vi "Aim Turret.vi"(0 "Setpoint (testing purposes only)":dbl, 1 "Goal Detected":bool=TRUE, 2 "Override?":bool, 3 "Override Setpoint":dbl, 4 "MotorControlDevRef":T2={"DeviceStatus"={"status"=FALSE, "code"=0, "source"=""}, "Type"=enum."CANTalonSRX", "PWM"={"PWM Channel"=enum."PWM 1", "DeadBand"={"Name"="", "maxPositivePwm"=0, "minPositivePwm"=0, "centerPwm"=0, "maxNegativePwm"=0, "minNegativePwm"=0, "angularRange"=0}}, "CAN"={"Device Number"=11, "Control Mode"=enum."Percent VBus", "Semaphore"=refnum, "Max Vout"=12.0, "TalonSRX Control Mode"=enum."Position"}, "Invert"=TRUE}, 5 "Goal Angle Degrees 0=straight ahead":dbl=0.37665367540620964, 6 "Yaw (degrees 0 = straight ahead gets larger clockwise)":dbl=-20.33, 7 "Sensor Position (degrees)":dbl=20.326171875, 9 "Softlimit":dbl=145.0 format="%#_13g") -> (14 "Output":dbl=20.702825550406203, 15 "Finished?":bool=TRUE, 18 "Override Still Enabled":bool)   [LabVIEW 2015]
uses:
  <vilib>/Rock Robotics/WPI/MotorControl/WPI_MotorControlDeviceRef.ctl
  <vilib>/Rock Robotics/WPI/MotorControl/WPI_MotorControlType.ctl
  <vilib>/Rock Robotics/SystemInterfaces/DIO/FPGA_DIOPWMChannel.ctl
  <vilib>/Rock Robotics/WPI/PWM/WPI_PWMDeadband.ctl
  <vilib>/Rock Robotics/WPI/CAN/Jaguar/SubVIs/WPI_CANJaguar_ControlMode.ctl
  <vilib>/Rock Robotics/WPI/CAN/TalonSRX/WPI_CANTalonSRX_APIControlMode.ctl
  Robot Global Data.vi
panel:
  in  "Turret PID (position) Long Distance Seek":T1={"P"=0.21, "I"=0.0021, "D"=3.0, "F"=0.0, "I Zone"=1200.0}
  in  "Turret PID (position) Short distance seek":T1={"P"=0.0015, "I"=0.0035, "D"=0.0, "F"=0.0, "I Zone"=1400.0}
  in  "Delay (ms)":i32=750
  in  "Turret revolutions per shooter revolution":dbl=15.0
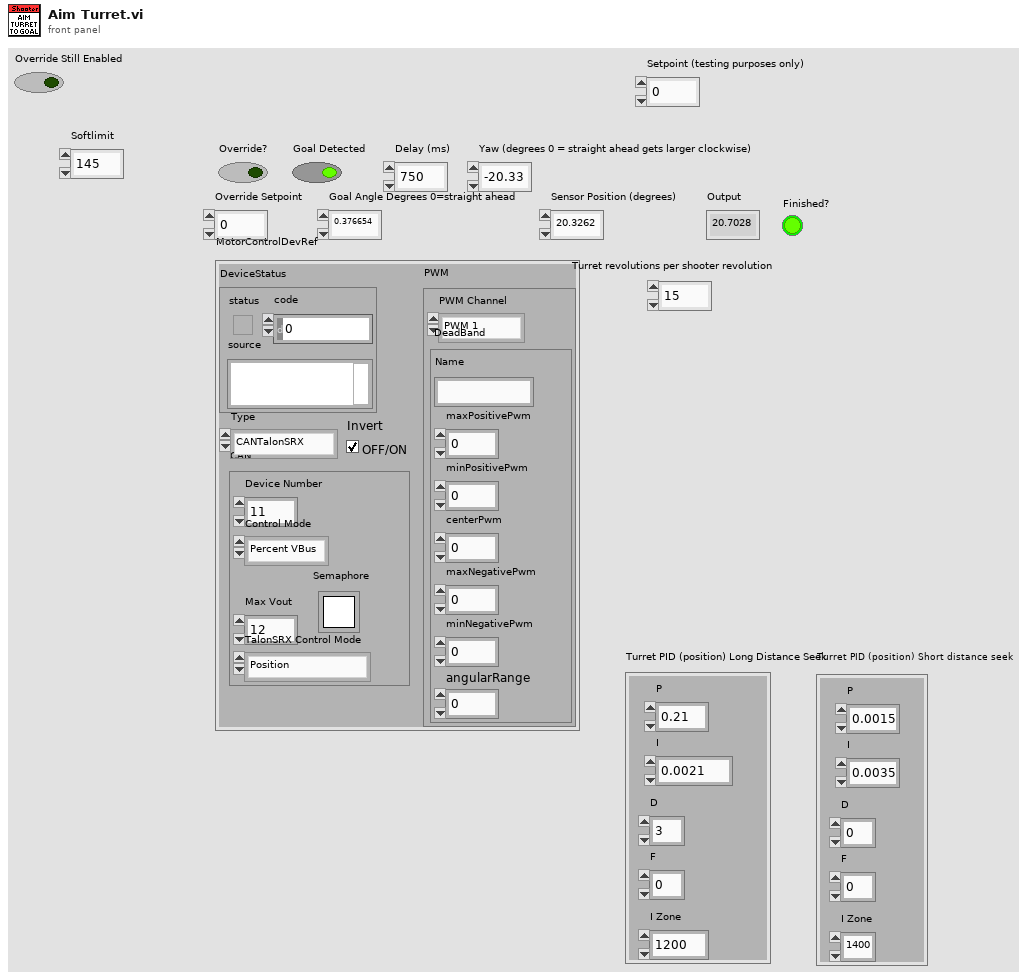
[diagram p1: front panel]
types:
  T1 = cluster{"P":dbl, "I":dbl, "D":dbl, "F":dbl, "I Zone":dbl}
  T2 = typedef "WPI_MotorControlDeviceRef.ctl" = cluster{"DeviceStatus":errorcluster, "Type":T3, "PWM":cluster{"PWM Channel":T4, "DeadBand":T5}, "CAN":cluster{"Device Number":u8, "Control Mode":T6, "Semaphore":T7, "Max Vout":dbl, "TalonSRX Control Mode":T8}, "Invert":bool}
  T3 = typedef "WPI_MotorControlType.ctl" = enum16{"PWM", "CAN", "CANTalonSRX"}
  T4 = typedef "FPGA_DIOPWMChannel.ctl" = enum8{"PWM 0", "PWM 1", "PWM 2", "PWM 3", "PWM 4", "PWM 5", "PWM 6", "PWM 7", "PWM 8", "PWM 9", "PWM MXP 0", "PWM MXP 1", "PWM MXP 2", "PWM MXP 3", "PWM MXP 4", "PWM MXP 5", "PWM MXP 6", "PWM MXP 7", "PWM MXP 8", "PWM MXP 9", "Invalid"}
  T5 = typedef "WPI_PWMDeadband.ctl" = cluster{"Name":string, "maxPositivePwm":i32, "minPositivePwm":i32, "centerPwm":i32, "maxNegativePwm":i32, "minNegativePwm":i32, "angularRange":u16}
  T6 = typedef "WPI_CANJaguar_ControlMode.ctl" = enum8{"Percent VBus", "Current", "Speed", "Position", "Voltage"}
  T7 = typedef "Semaphore RefNum" = refnum<k1>
  T8 = typedef "WPI_CANTalonSRX_APIControlMode.ctl" = enum8{"Percent VBus", "Speed", "Position", "Slave", "Unchanged / Invalid", "Voltage Compensation", "Current", "Motion Profile"}
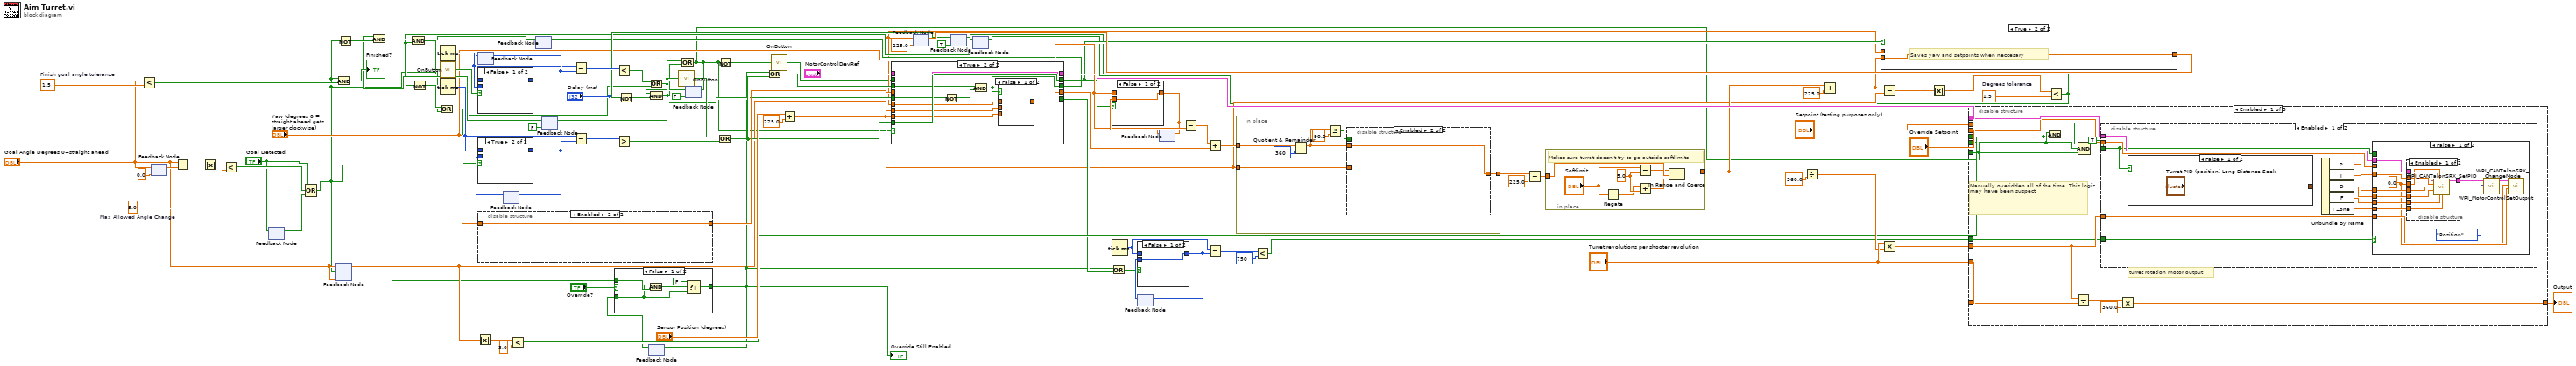
[diagram p0: block diagram]
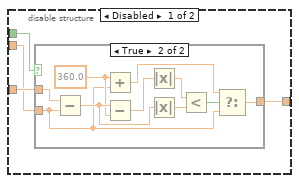
[diagram p4: hidden frame]
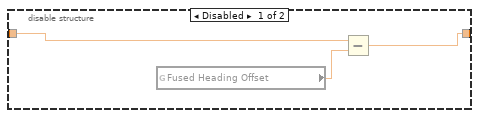
[diagram p6: hidden frame]
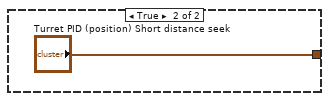
[diagram p10: hidden frame]
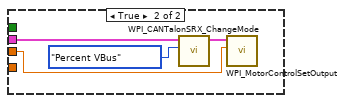
[diagram p12: hidden frame]
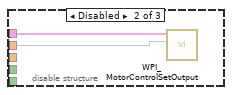
[diagram p14: hidden frame]
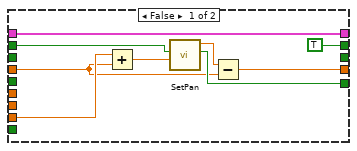
[diagram p17: hidden frame]
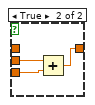
[diagram p18: hidden frame]
diagram:
  w11 = 5.0  # Max Allowed Angle Change
  w44 = 1.5  # Degrees tolerance
  w86 = 1.5  # Finish goal angle tolerance
  n1 = Less?(x="Goal Angle Degrees 0=straight ahead", y=w86) -> (x < y?=w85:bool)
  n2 = feedback-in #1("Goal Angle Degrees 0=straight ahead") -> ()
  n3 = feedback #1(0.0 ("Goal Angle Degrees 0=straight ahead")) -> (w15:dbl)
  n4 = Subtract(x="Goal Angle Degrees 0=straight ahead", y=w15) -> (x-y=w13:dbl)
  n5 = Absolute Value(x=w13) -> (abs(x)=w12:dbl)
  n6 = Less?(x=w12, y=w11) -> (x < y?=w4:bool)
  n7 = feedback-in #2("Goal Detected") -> ()
  n8 = feedback #2() -> (w5:bool)  [unwired: 1 in]
  n9 = Compound Arithmetic op=OR("Goal Detected", w4, w5) -> (w2:bool)
  n10 = feedback-in #3("Goal Angle Degrees 0=straight ahead", w2) -> ()
  n11 = feedback #3("Goal Angle Degrees 0=straight ahead") -> (w9:dbl)
  n12 = Not(x=w2) -> (.not. x?=w70:bool)
  n13 = Compound Arithmetic op=AND(w2, w85) -> (→"Finished?":bool)
  n14 = Tick Count (ms)() -> (millisecond timer value=w73:u32)
  n15 = Tick Count (ms)() -> (millisecond timer value=w79:u32)
  n16 = Absolute Value(x=w9) -> (abs(x)=w16:dbl)
  n17 = feedback #4() -> (w75:u32)  [unwired: 1 in]
  n18 = disable-structure shown="Enabled" {
    disable-tunnel: [w99 w100] -> w89
    disable-tunnel: "Yaw (degrees 0 = straight ahead gets larger clockwise)" -> [w97 w100]
    frame Disabled {
      n19 = global read "Robot Global Data.vi" "Fused Heading Offset"() -> (w98:dbl)
      n20 = Subtract(x=w97, y=w98) -> (x-y=w99:dbl)
    }
    frame Enabled {
    }
  }
  n21 = feedback #5() -> (w82:u32)  [unwired: 1 in]
  n22 = Less?(x=w16, y=3.0 ("x")) -> (x < y?=w31:bool)
  n23 = feedback #6() -> (w37:bool)  [unwired: 1 in]
  n24 = feedback #7(FALSE) -> (w69:bool)
  n25 = And(x=w69, y=w70) -> (x .and. y?=w68:bool)
  n26 = feedback #8() -> (w8:bool)  [unwired: 1 in]
  n27 = case shown="False" "Override?" {
    selector: "Override?" -> [_ w106]
    tunnel: [w101 w106] -> w6
    tunnel: w8 -> [w102 _]
    tunnel: w2 -> [w105 _]
    frame False {
      n28 = And(x=w102, y=w105) -> (x .and. y?=w104:bool)
      n29 = Select(t=FALSE, s=w104, f=w102) -> (s? t:f=w101:bool)
    }
    frame True {
    }
  }
  "Override Still Enabled" <- w6
  n30 = feedback-in #8(w6) -> ()
  n31 = feedback #9(FALSE) -> (w63:bool)
  n32 = Add(x="Sensor Position (degrees)", y=225.0) -> (x+y=w18:dbl)
  n33 = feedback #10(225.0) -> (w32:dbl)
  n34 = feedback #11(TRUE) -> (w64:bool)
  n35 = Not(x=w64) -> (.not. x?=w78:bool)
  n36 = And(x=w63, y=w78) -> (x .and. y?=w42:bool)
  n37 = feedback #12() -> (w40:bool)  [unwired: 1 in]
  n38 = And(x=w68, y=w40) -> (x .and. y?=w66:bool)
  n39 = Not(x=w40) -> (.not. x?=w39:bool)
  n40 = Or(x=w39, y=w37) -> (x .or. y?=w38:bool)
  n41 = call "OnButton.vi"("Button"=w66) -> ("Value"=w65:bool)  [unwired: 1 in]
  n42 = case shown="False" w65 {
    tunnel: [w107 w108] -> w74
    tunnel: w73 -> [_ w108]
    tunnel: w75 -> [w107 _]
    frame False {
    }
    frame True {
    }
  }
  n43 = feedback-in #4(w74) -> ()
  n44 = case shown="True" w38 {
    tunnel: [w109 w110] -> w81
    tunnel: w79 -> [_ w110]
    tunnel: w82 -> [w109 _]
    frame False {
    }
    frame True {
    }
  }
  n45 = feedback-in #5(w81) -> ()
  n46 = Subtract(x=w73, y=w74) -> (x-y=w76:u32)
  n47 = Subtract(x=w79, y=w81) -> (x-y=w83:u32)
  n48 = Less?(x=w76, y="Delay (ms)") -> (x < y?=w72:bool)
  n49 = Greater?(x=w83, y="Delay (ms)") -> (0:w80:bool)
  n50 = Or(x=w72, y=w2) -> (x .or. y?=w71:bool)
  n51 = feedback-in #7(w71) -> ()
  n52 = call "OnButton.vi"("Button"=w71) -> ("Value"=w77:bool)  [unwired: 1 in]
  n53 = Or(x=w71, y=w42) -> (x .or. y?=w1:bool)
  n54 = feedback-in #9(w1) -> ()
  n55 = Or(x=w77, y=w80) -> (x .or. y?=w52:bool)
  n56 = Not(x=w1) -> (.not. x?=w21:bool)
  n57 = Or(x=w6, y=w52) -> (x .or. y?=w57:bool)
  n58 = call "OnButton.vi"("Button"=w21) -> ("Value"=w20:bool)  [unwired: 1 in]
  n59 = case shown="True" w1 {
    tunnel: "MotorControlDevRef" -> [w119 w129]
    tunnel: [w119 w129] -> w90
    tunnel: w9 -> [_ w126]
    tunnel: [TRUE w128] -> w53
    tunnel: w52 -> [_ w128]
    tunnel: [w115 w125] -> w87
    tunnel: w18 -> [w113 w127]
    tunnel: w89 -> [w111 _]
    tunnel: w57 -> [_ w123]
    tunnel: w32 -> [_ w124]
    tunnel: w42 -> [_ w121]
    tunnel: [_ w120] -> w41
    tunnel: [w116 _] -> w22
    tunnel: w20 -> [w117 _]
    frame False {
      n60 = Add(x=w113, y=w111) -> (x+y=w112:dbl)
      n61 = call "SetPan.vi"("Sensor Position"=w112, "New Command"=w117) -> ("Reached Setpoint"=w116:bool, "Pan Setpoint"=w118:dbl)  [unwired: 8 in]
      n62 = Subtract(x=w118, y=w111) -> (x-y=w115:dbl)
    }
    frame True {
      n63 = Not(x=w121) -> (.not. x?=w122:bool)
      n64 = And(x=w123, y=w122) -> (x .and. y?=w120:bool)
      n65 = case shown="False" w120 {
        tunnel: w127 -> [_ w133]
        tunnel: w126 -> [_ w132]
        tunnel: [w130 w131] -> w125
        tunnel: w124 -> [w130 _]
        frame False {
        }
        frame True {
          n66 = Add(x=w132, y=w133) -> (x+y=w131:dbl)
        }
      }
    }
  }
  n67 = feedback-in #6(w41) -> ()
  n68 = Or(x=w6, y=w22) -> (x .or. y?=w23:bool)
  n69 = Tick Count (ms)() -> (millisecond timer value=w28:u32)
  n70 = feedback #13() -> (w30:u32)  [unwired: 1 in]
  n71 = case shown="False" w23 {
    tunnel: [w134 w135] -> w29
    tunnel: w28 -> [_ w135]
    tunnel: w30 -> [w134 _]
    frame False {
    }
    frame True {
    }
  }
  n72 = feedback-in #13(w29) -> ()
  n73 = feedback #14() -> (w56:dbl)  [unwired: 1 in]
  n74 = case shown="False" w53 {
    tunnel: [w136 w137] -> w54
    tunnel: w56 -> [w136 _]
    tunnel: "Yaw (degrees 0 = straight ahead gets larger clockwise)" -> [_ w137]
    frame False {
    }
    frame True {
    }
  }
  n75 = feedback-in #14(w54) -> ()
  n76 = Subtract(x=w54, y="Yaw (degrees 0 = straight ahead gets larger clockwise)") -> (x-y=w51:dbl)
  n77 = Add(x=w51, y=w87) -> (x+y=w33:dbl)
  n78 = Subtract(x=w28, y=w29) -> (x-y=w25:u32)
  n79 = in-place {
    in-place-border: w18 -> [w142]
    in-place-border: [w141] -> w47
    in-place-border: w33 -> [w140]
    n80 = Quotient & Remainder(x=w140, y=360) -> (x-y*floor(x/y)=w138:dbl)  [unwired: 1 out]
    n81 = Less Or Equal?(x=w138, y=90.0) -> (x <= y?=w143:bool)
    n82 = disable-structure shown="Enabled" {
      disable-tunnel: w143 -> [w148 _]
      disable-tunnel: w142 -> [w147 _]
      disable-tunnel: [w146 w160] -> w141
      disable-tunnel: w138 -> [w145 w160]
      frame Disabled {
        n83 = case shown="True" w148 {
          tunnel: [w149 w150] -> w146
          tunnel: w145 -> [w149 w151]
          tunnel: w147 -> [_ w155]
          frame False {
          }
          frame True {
            w153 = 360.0 ("y")
            n84 = Subtract(x=w155, y=w151) -> (x-y=w154:dbl)
            n85 = Add(x=w153, y=w151) -> (x+y=w152:dbl)
            n86 = Subtract(x=w154, y=w153) -> (x-y=w159:dbl)
            n87 = Absolute Value(x=w159) -> (abs(x)=w158:dbl)
            n88 = Absolute Value(x=w154) -> (abs(x)=w157:dbl)
            n89 = Less?(x=w158, y=w157) -> (x < y?=w156:bool)
            n90 = Select(t=w152, s=w156, f=w151) -> (s? t:f=w150:dbl)
          }
        }
      }
      frame Enabled {
      }
    }
  }
  n91 = Less?(x=w25, y=u32 750 ("x")) -> (x < y?=w27:bool)
  n92 = Subtract(x=w47, y=225.0) -> (x-y=w19:dbl)
  n93 = in-place {
    in-place-border: w19 -> [w167]
    in-place-border: [w166] -> w36
    w164 = 5.0 ("y")
    # "Makes sure turret doesn't try to go outside softlimits"
    n94 = Negate(x="Softlimit") -> (-x=w162:dbl)
    n95 = Subtract(x="Softlimit", y=w164) -> (x-y=w165:dbl)
    n96 = Add(x=w162, y=w164) -> (x+y=w163:dbl)
    n97 = In Range and Coerce(upper limit=w165, x=w167, lower limit=w163) -> (coerced(x)=w166:dbl)  [unwired: 1 out]
  }
  n98 = Divide(x=w36, y=360.0) -> (x/y=w50:dbl)
  n99 = Add(x=w36, y=225.0) -> (x+y=w35:dbl)
  n100 = case shown="True" w53 {
    tunnel: [w168 w169] -> w95
    tunnel: w35 -> [_ w169]
    tunnel: w32 -> [w168 _]
    frame False {
      # "Saves yaw and setpoints when neccesary"
    }
    frame True {
      # "Saves yaw and setpoints when neccesary"
    }
  }
  n101 = feedback-in #10(w95) -> ()
  n102 = Subtract(x=w35, y=w18) -> (x-y=w46:dbl)
  n103 = Multiply(x="Turret revolutions per shooter revolution", y=w50) -> (x*y=w94:dbl)
  n104 = Absolute Value(x=w46) -> (abs(x)=w45:dbl)
  n105 = disable-structure shown="Enabled" {
    disable-tunnel: w94 -> [w179 _ _]
    disable-tunnel: "Turret revolutions per shooter revolution" -> [_ _ _]
    disable-tunnel: "Setpoint (testing purposes only)" -> [_ w220 _]
    disable-tunnel: "Turret revolutions per shooter revolution" -> [w178 _ _]
    disable-tunnel: [w177 _ _] -> w91
    disable-tunnel: w90 -> [w176 w219 _]
    disable-tunnel: "Override Setpoint" -> [w175 _ _]
    disable-tunnel: w31 -> [w171 _ _]
    disable-tunnel: w27 -> [w174 _ _]
    disable-tunnel: w1 -> [w173 _ _]
    disable-tunnel: w1 -> [w172 _ _]
    frame Enabled {
      # "Manuelly overidden all of the time. This logic may have been suspect"
      # "turret rotation motor output"
      n106 = And(x=w173, y=w171) -> ()  [unwired: 1 out]
      n107 = Divide(x=w179, y=w178) -> (x/y=w180:dbl)
      n108 = Compound Arithmetic op=AND(w171, w173, w172) -> ()  [unwired: 1 out]
      n109 = disable-structure shown="Enabled" {
        disable-tunnel: w179 -> [w192 _]
        disable-tunnel: w176 -> [w189 _]
        disable-tunnel: w175 -> [w191 _]
        disable-tunnel: TRUE -> [w182 _]
        disable-tunnel: w174 -> [w190 _]
        frame Enabled {
          n110 = case shown="False" w182 {
            tunnel: ["Turret PID (position) Long Distance Seek" "Turret PID (position) Short distance seek"] -> w188
            frame False {
            }
            frame True {
            }
          }
          n111 = Unbundle By Name(w188) -> ("P"=w187:dbl, "I"=w186:dbl, "D"=w185:dbl, "F"=w183:dbl, "I Zone"=w184:dbl)
          n112 = case shown="False" w190 {
            tunnel: w192 -> [w205 _]
            tunnel: w191 -> [_ w218]
            tunnel: w189 -> [w202 w215]
            tunnel: w187 -> [w200 _]
            tunnel: w186 -> [w199 _]
            tunnel: w185 -> [w198 _]
            tunnel: w184 -> [w197 _]
            tunnel: w183 -> [w196 _]
            tunnel: w182 -> [_ _]
            frame False {
              w195 = 0.0
              n113 = disable-structure shown="Enabled" {
                disable-tunnel: w202 -> [w213 w214]
                disable-tunnel: [w212 w214] -> w201
                disable-tunnel: w195 -> [w211 _]
                disable-tunnel: w200 -> [w210 _]
                disable-tunnel: w199 -> [w209 _]
                disable-tunnel: w198 -> [w208 _]
                disable-tunnel: w197 -> [w207 _]
                disable-tunnel: w196 -> [w206 _]
                frame Enabled {
                  n114 = call <vilib>:"WPI_CANTalonSRX_SetPID.vi"("CAN Talon SRX Ref"=w213, "Parameter Slot"=w211, "P"=w210, "I"=w209, "D"=w208, "F"=w206, "I Zone"=w207) -> ("CAN Talon SRX Ref"=w212:T2)  [unwired: 7 in, 1 out]
                }
                frame Disabled {
                }
              }
              n115 = call <vilib>:"WPI_CANTalonSRX_ChangeMode.vi"("Control Mode"=WPI_CANTalonSRX_APIControlMode."Position", "CAN Talon SRX Ref"=w201) -> ("CAN Talon SRX Ref"=w203:T2)  [unwired: 8 in, 1 out]
              n116 = call <vilib>:"WPI_MotorControlSetOutput.vi"("Sync Group / Parameter Slot"=w195, "Output"=w205, "MotorControlDevRef"=w203) -> ()  [unwired: 6 in, 3 out]
            }
            frame True {
              n117 = call <vilib>:"WPI_CANTalonSRX_ChangeMode.vi"("Control Mode"=WPI_CANTalonSRX_APIControlMode."Percent VBus", "CAN Talon SRX Ref"=w215) -> ("CAN Talon SRX Ref"=w217:T2)  [unwired: 8 in, 1 out]
              n118 = call <vilib>:"WPI_MotorControlSetOutput.vi"("Output"=w218, "MotorControlDevRef"=w217) -> ()  [unwired: 7 in, 3 out]
            }
          }
        }
        frame Disabled {
        }
      }
      n119 = Multiply(x=w180, y=360.0) -> (x*y=w177:dbl)
    }
    frame Disabled {
      n120 = call <vilib>:"WPI_MotorControlSetOutput.vi"("Output"=w220, "MotorControlDevRef"=w219) -> ()  [unwired: 7 in, 3 out]
    }
    frame Disabled {
    }
  }
  "Output" <- w91
  n121 = Less?(x=w45, y=w44) -> (x < y?=w17:bool)
  n122 = feedback-in #11(w17) -> ()
  n123 = feedback-in #12(w17) -> ()
